vi "Big_LED_control.vi"() -> ()   [LabVIEW 2018]
uses:
  <instrlib>/niDCPower/nidcpower.llb/niDCPower Source Mode.ctl
  <instrlib>/niDCPower/nidcpower.llb/niDCPower Output Function.ctl
  AT lib/AmateurStepperMotor.dll
  <instrlib>/niDMM/nidmm.llb/niDMM Function.ctl
  <instrlib>/niDMM/nidmm.llb/niDMM Resolution in Digits.ctl
  <vilib>/Instr/_visa.llb/VISA Configure Serial Port (Instr).vi
  <instrlib>/niDMM/nidmm.llb/niDMM Configure Measurement Digits.vi
panel:
  in  "Go To 2":dbl
  in  "Погнали! 2":bool
  in  "HoldOn 2":bool
  in  "Tab Control 2":enum32{"Шаговик и офир", "Служебная область"}(tab)
  in  "milliseconds to wait":u32=1000
  in  "Go To":dbl
  out "Ophir 1 Char":dbl(graph)=0.02
  in  "DecelerationTime, s":dbl=0.3
  in  "AccelerationTime, s":dbl=0.3
  in  "HoldOn":bool
  in  "Ophir 1 units":string(combo)="1000" caption="Units"
  out "Ophir 1 Over Range":bool caption="Over Range"
  out "Ophir 1 Optical Power":dbl=0.02 caption="Power" format="%#_4g"
  out "Ophir 1 MAX":dbl=0.030000000000000002 caption="MAX" format="%#_5g"
  in  "Ophir 1 Clear":bool caption="Clear"
  in  "StepMultiplicationFactor":dbl=50.0
  in  "StepDivisor":i32(ring)=8 items=["D1"=1, "D2"=2, "D4"=4, "D8"=8, "D16"=16, "D32"=32]
  in  "Speed":dbl=250.0
  in  "Погнали!":bool
  in  "Стоп GoTo":bool
  out "Готово":bool
  out "Position":dbl
  in  "Ophir 1 Info":u16(ring)=1 caption="Info" items=["Device : JUNO; s/n:903793", "Head : PD300R-3W   ; s/n:779628"]
  in  "new pos":dbl
  in  "set pos":bool
  out "Device Response":string="*\n"
  in  "Ophir 1 usb channel":i16 caption="usb channel"
  out "Ophir 1 dup Visa Session":refnum<visa-resource-name>="USB0::0x0BD3::0x0777::NI-VISA-60004::RAW" caption="dup Visa Session"
  in  "Ophir 1 Baud Rate (3:9600)":i16(ring)=3 caption="Baud Rate (3:9600)" items=["300", "1200", "4800", "9600", "19200", "38400"]
  out "Ophir 1 Real Optical Power":dbl=2e-05 format="%.6e"
  in  "Ophir 1 GPIB Address (10)":string="10" caption="GPIB Address (10)"
  in  "Ophir 1 Port Number (default 2)":i16=1 caption="Port Number (default 2)" min=0 max=20
  in  "Ophir 1 Select Communication Protocol":u16(ring) caption="Select Communication Protocol" items=["USB", "RS232", "GPIB"]
  out "Ophir 1 error out":errorcluster caption="error out"
  in  "Ophir 1 error in (no error)":errorcluster caption="error in (no error)"
  in  "Ophir 1 Wait":u32=100 caption="Wait"
  out "IsOpen":bool=TRUE
  out "Ophir 1 Initialization":bool=TRUE caption="Initialization"
  in  "Tab Control":T1(tab)
  in  "POWER":bool
  in  "Стоп":bool=TRUE
  in  "Resource Name":refnum<k15>="PXI1Slot2" caption="Источник питания"
  in  "Амперметр":refnum<k15>="PXI1Slot4" caption="NI DMM 1"
  in  "V_MB, V":dbl=2.0 caption="voltage level" format="%_6p"
  in  "curlim_V_MB, A":dbl=0.3 caption="current limit" format="%_6p"
  out "chart_0":dbl(graph)=-0.00019003121552656476 caption="Waveform Chart 5"
  in  "voltlim_I_LED, V":dbl=2.0 caption="current limit" min=0.01 format="%_6p"
  in  "I_LED, A":dbl=0.005 caption="voltage level" format="%_6p"
  out "chart_1":dbl(graph)=-0.00011794146773492402 caption="Waveform Chart 5"
  out "Current Char":dbl(graph)=0.004513189196586609
  in  "Arduino":refnum<visa-resource-name>="COM14"
  in  "Сегменты":bool[](array[boolean])=[FALSE, FALSE, FALSE, FALSE, FALSE, FALSE, FALSE, FALSE, FALSE, FALSE, FALSE, FALSE, FALSE, FALSE, FALSE, FALSE, FALSE, FALSE]
  in  "Вольтметр":refnum<k15>="PXI1Slot5" caption="NI DMM 1"
  out "Voltage Char":dbl(graph)=0.015767553821206093
  in  "Port Name":string="COM4" caption="Порт шаговика"
  in  "wave_lenght":string="600"
  in  "Промер":bool caption="Промер сегмента"
  in  "NI DMM 1 Voltage Range 4":string(combo)="-1" caption="Range"
  in  "NI DMM 1 units 4":string(combo)="1" caption="Units"
  out "Voltage":dbl=0.015767553821206093 format="%_6g"
  in  "NI DMM 1 Current Range 3":string(combo)="1" caption="Range"
  in  "NI DMM 1 units 3":string(combo)="1000" caption="Units"
  out "Current":dbl=0.004513189196586609 format="%_6g"
  out "voltmes_V_MB, V":dbl=-0.00019003121552656476 caption="measurement" format="%_6g"
  out "curmes_V_MB, A":dbl=4.978853713564661e-05 caption="measurement" format="%_6g"
  out "curmes_I_LED, A":dbl=4.978853713564661e-05 caption="measurement" format="%_6g"
  out "voltmes_I_LED, V":dbl=-0.00011794146773492402 caption="measurement" format="%_6g"
  out "Разряд":dbl
  out "+/-":bool
  out "Power off":bool=TRUE
  in  "Command":string="Cathode"
  in  "Записать":bool
  out "measure output file refnum":refnum<file>
  out "Voltage, V":dbl=0.015767553821206093 caption="Measurement" format="%.5f"
  out "Current, A":dbl=4.513189196586609e-06 caption="Measurement" format="%.5f"
  out "Тип индикатора":string="Cathode"
  out "chart_2":dbl(graph)=-0.000179732680132088
  in  "V_RES, V":dbl caption="voltage level" format="%_6p"
  out "curmes_V_RES, A":dbl=5.996099535583298e-05 caption="measurement" format="%_6g"
  in  "curlim_V_RES, A":dbl=0.1 caption="current limit" min=0.01 format="%_6p"
  in  "measure path":path=path "D:/NI LabVIEW/MultiOpto/MultiOpto_1.2/Logs/SEL"
  out "Enum":enum16{"Exit", "4", "Промер", "2", "1"}(ring)
  out "№ об-ца":dbl=1.0
  out "Темп-ра":dbl=1.0
  out "Сегмент":string
  out "voltmes_V_RES, V":dbl=-0.000179732680132088 caption="measurement" format="%_6g"
  in  "current level range":dbl=0.001 format="%#.6p"
  # "Шаговик"
  # "Офир"
  # "Шаговик"
  # "Офир"
  # "position - это значение абсолютное"
  # "j"
  # "c"
  # "d"
  # "e"
  # "g"
  # "h"
  # "a"
  # "b"
  # "f"
  # "k"
  # "L"
  # "m"
  # "n"
  # "p"
  # "dp"
  # "all"
  # "V_MB 5 В\nогрничение 300 м\n\nV_LED 2,1 В\nограничение 200 м"
  # "единицы мА\nrange 1 А"
  # "1. каждый сегмент включаем по отдельности, резистором постраиваем ток до 10 мА\n2. напряжение V_LED при этом не меняется\n3. в такоом положении промеряем сегменты по отдельности\n4. для промера всего индикатора сразу подстраиваем напряжение при неизменном положении резисторов\n5. ток всех индикаторов = ток одного сегмента (10 мА) * число сегментов (15)\n6. добиваемся этого увеличением V_LED"
  # "единицы В\nrange AUTO"
  # "регклировка суммарного тока через индикатор"
  # "24.063\n\n     I          U\n20 мА  1.3 В\n20 мА  1.4 В\n 7 мА   1.15 В"
  # "24.064\n\n     I          U\n10 мА  2 В\n10 мА  2.15 В\n 7 мА   1.9 В"
  # "автоматизировать подбор напряжения по известному максимальному напряжению и току. ОС по току сегмента"
  # "Р1:  +25°C\nР2:  - 60°C\nР3:  +85°C"
  # "регулировать ток в зависимости от температуры.\nс ростом температуры растет ток.\nпид-регулятор??"
  # "0. ввести номер образца\n1. включить нужный сегмент\n2. ввести его в поле справа\n3. вести температуру в поле слева\n4. нажать кнопку \"промер сегмента\""
  # "\"опрашивать кнопки не чаще, чем раз в секунду. сейчас кликать можно чаще, они загорятся, но ничего не произойдет\""
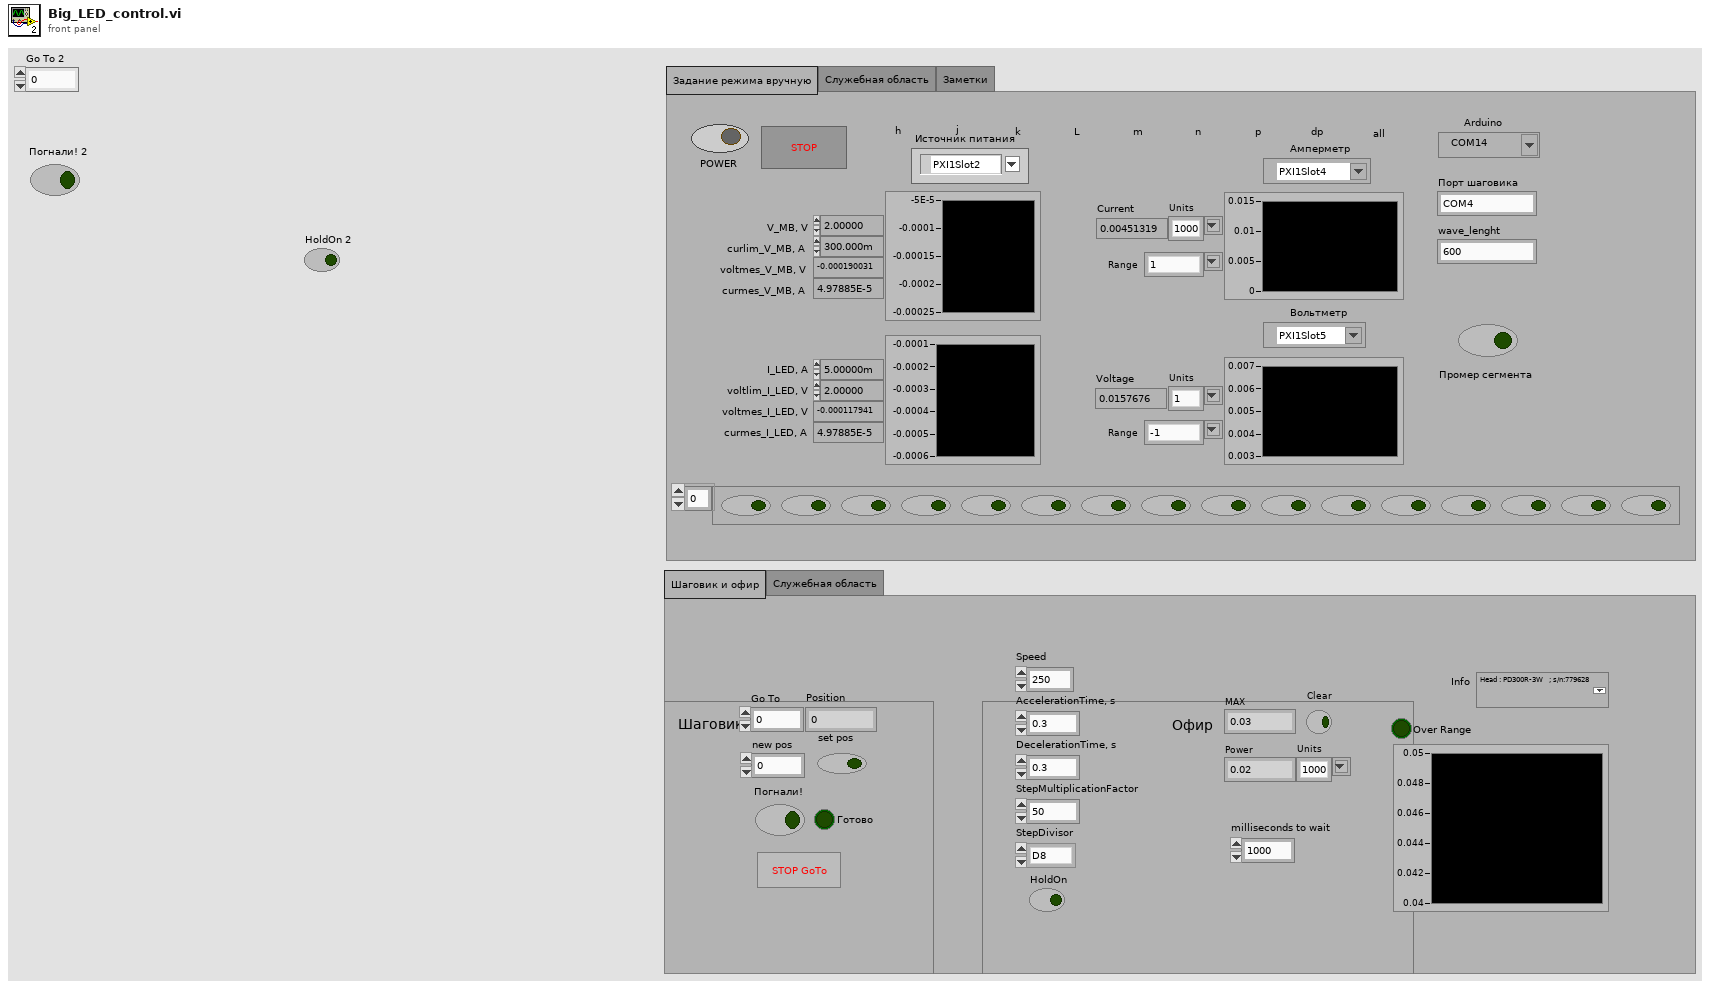
[diagram p1: front panel]
types:
  T1 = enum32{"Задание режима вручную", "Служебная область", "Заметки"}
  T2 = enum16{"open", "replace", "create", "open or create", "replace or create", "replace or create with confirmation"}
  T3 = typedef "niDCPower Output Function.ctl" = i32
  T4 = typedef "niDCPower Source Mode.ctl" = i32
  T5 = typedef "niDMM Function.ctl" = enum16{"DC Volts", "AC Volts", "DC Current", "AC Current", "2-wire Resistance", "4-wire Resistance", "Diode", "Frequency", "Period", "AC Volts DC Coupled", "Capacitance", "Inductance", "Temperature"}
  T6 = typedef "niDMM Resolution in Digits.ctl" = dbl
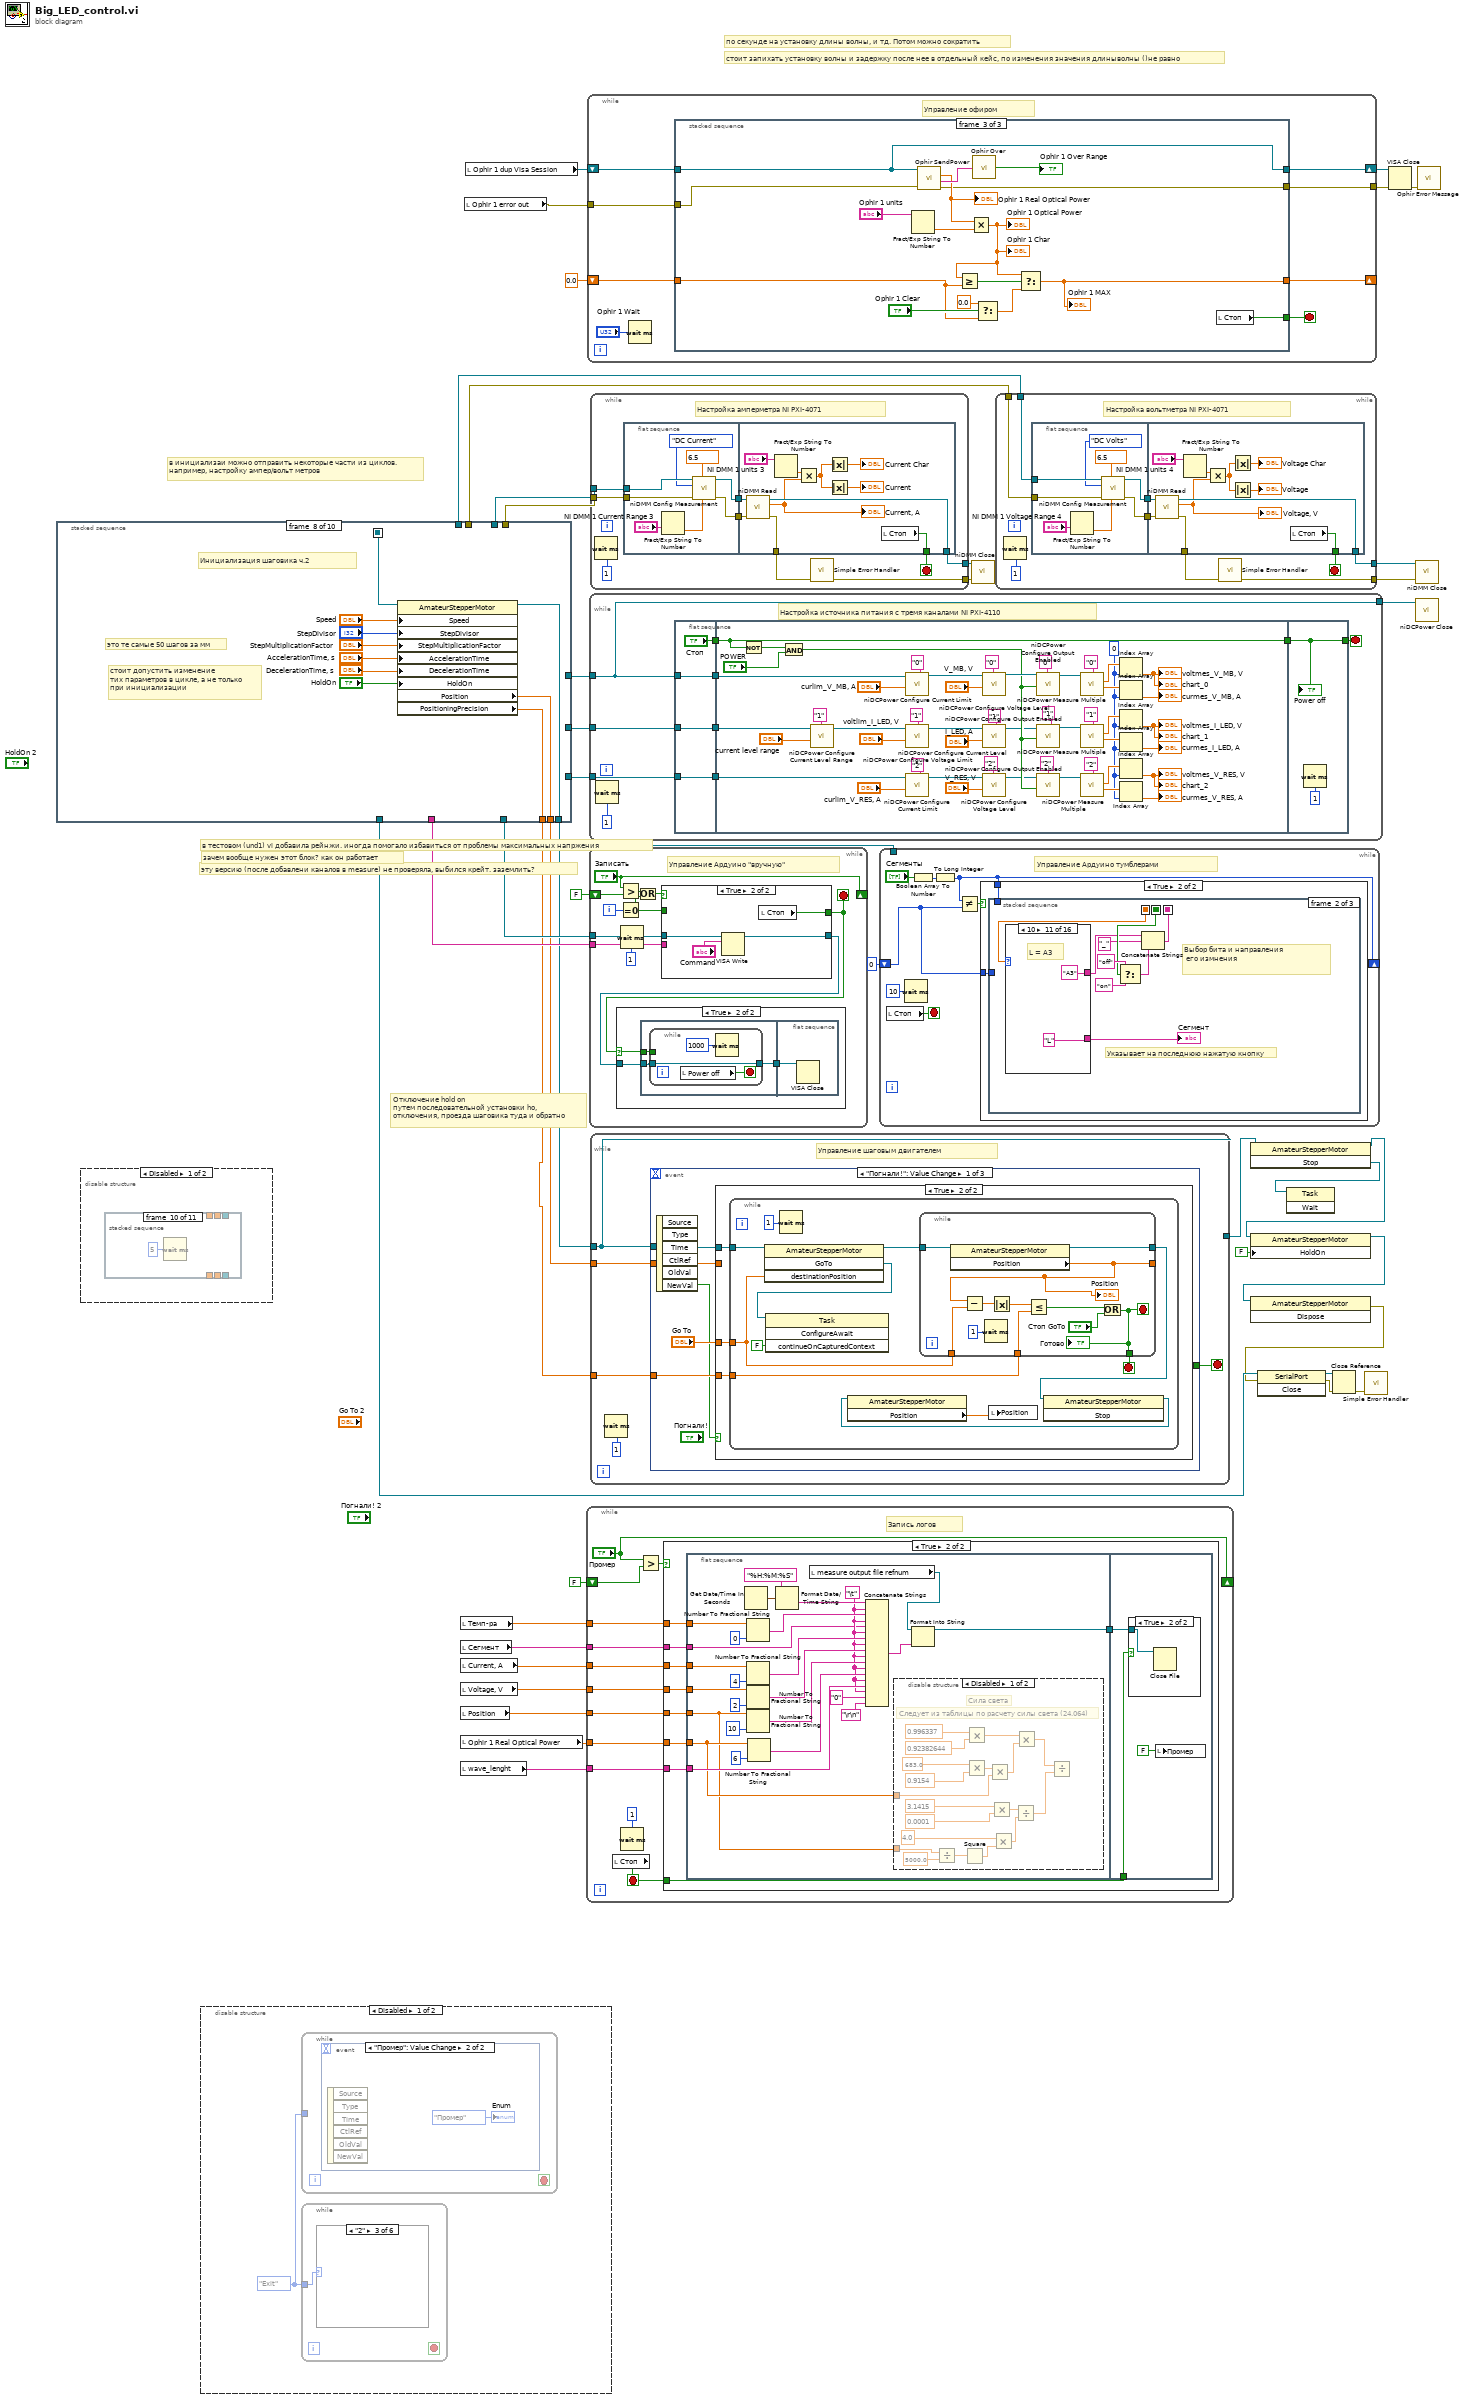
[diagram p0: block diagram]
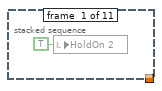
[diagram p2: hidden frame]
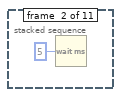
[diagram p3: hidden frame]
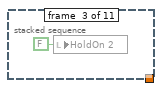
[diagram p4: hidden frame]
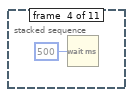
[diagram p5: hidden frame]
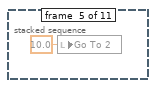
[diagram p6: hidden frame]
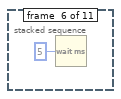
[diagram p7: hidden frame]
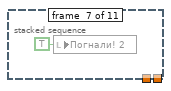
[diagram p8: hidden frame]
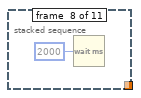
[diagram p9: hidden frame]
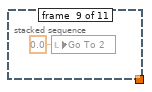
[diagram p10: hidden frame]
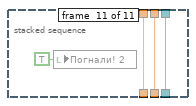
[diagram p11: hidden frame]
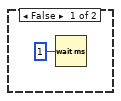
[diagram p13: hidden frame]
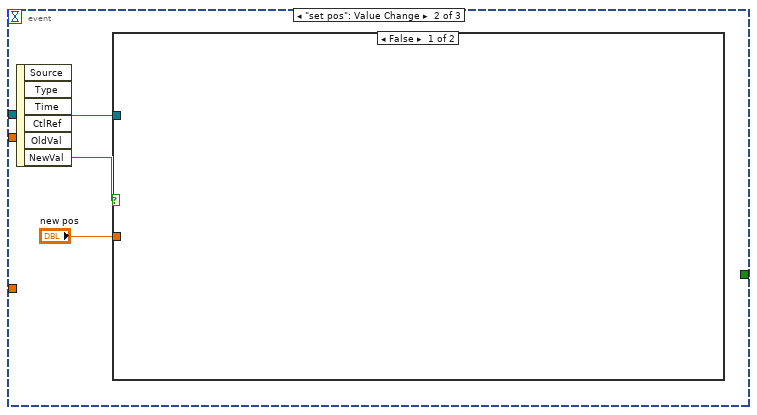
[diagram p14: hidden frame]
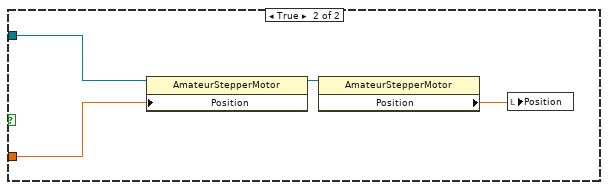
[diagram p15: hidden frame]
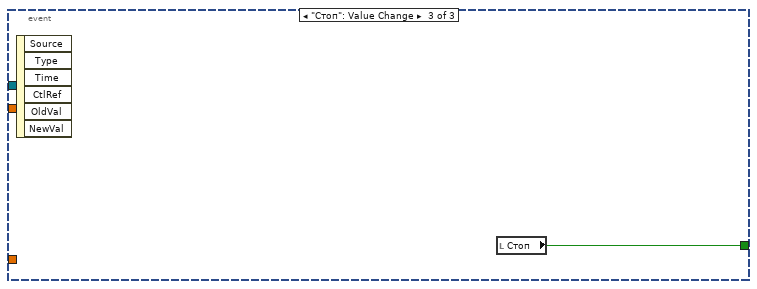
[diagram p16: hidden frame]
diagram:
  # "эту версию (после добавлени каналов в measure) не проверяла, выбился крейт. заземлить?"
  # "зачем вообще нужен этот блок? как он работает"
  # "в тестовом (und1) vi добавила рейнжи. иногда помогало избавиться от проблемы максимальных напржения"
  # "Отключение hold on\nпутем последовательной установки ho, \nотключения, проезда шаговика туда и обратно"
  # "в инициализаи можно отправить некоторые части из циклов.\nнапример, настройку ампер/вольт метров"
  # "стоит запихать установку волны и задержку после нее в отдельный кейс, по изменения значения длиныволны ()не равно"
  # "по секунде на установку длины волны, и тд. Потом можно сократить"
  n1 = stacked-sequence {
    seq-local: [_ _ _ _ _ _ w114 _ _ _] -> [_ _ _ _ _ _ _ w123 _ _]
    tunnel: [_ _ _ w61 _ _ _ _ _ _] -> w31
    tunnel: [_ w55 _ _ _ _ _ _ _ _] -> w43
    tunnel: [_ w54 _ _ _ _ _ _ _ _] -> w42
    tunnel: [_ _ _ _ w81 _ _ _ _ _] -> w39
    tunnel: [_ _ _ _ _ _ _ _ _ w161] -> w38
    tunnel: [_ _ w58 _ _ _ _ _ _ _] -> w37
    tunnel: [_ _ w57 _ _ _ _ _ _ _] -> w36
    tunnel: [_ _ _ _ _ _ _ w126 _ _] -> w1
    tunnel: [_ _ _ _ _ _ _ w124 _ _] -> w2
    tunnel: [_ _ _ _ _ _ _ w125 _ _] -> w3
    tunnel: [_ _ _ _ _ _ w104 _ _ _] -> w25
    tunnel: [_ _ _ w60 _ _ _ _ _ _] -> w8
    tunnel: [_ _ _ w59 _ _ _ _ _ _] -> w4
    frame #0 {
      w49 = 0.0 ("currentmes_2")
      w50 = FALSE ("Стоп")
      # "ch 1"
      # "Обнуление переменных"
      n2 = local write "POWER"(w50) -> ()
      n3 = local write "Стоп"(w50) -> ()
      n4 = local write "+/-"(w50) -> ()
      n5 = local write "Погнали!"(w50) -> ()
      n6 = local write "Готово"(w50) -> ()
      n7 = local write "Стоп GoTo"(w50) -> ()
      n8 = local write "Speed"(250.0 ("Speed")) -> ()
      n9 = local write "StepMultiplicationFactor"(50.0 ("StepMultiplicationFactor")) -> ()
      n10 = local write "AccelerationTime, s"(0.3 ("AccelerationTime, s")) -> ()
      n11 = local write "DecelerationTime, s"(0.3 ("DecelerationTime, s")) -> ()
      n12 = local write "Go To"(w49) -> ()
      n13 = local write "curmes_V_MB, A"(w49) -> ()
      n14 = local write "curmes_V_RES, A"(w49) -> ()
      n15 = local write "Current"(w49) -> ()
      n16 = local write "Разряд"(w49) -> ()
      n17 = local write "voltmes_I_LED, V"(w49) -> ()
      n18 = local write "Сегменты"(bool[] [FALSE, FALSE, FALSE, FALSE, FALSE, FALSE, FALSE, FALSE, FALSE, FALSE, FALSE, FALSE, FALSE, FALSE, FALSE, FALSE, FALSE, FALSE] ("Сегменты")) -> ()
      n19 = local write "current level range"(0.001 ("current level range")) -> ()
      n20 = local write "Command"("zero" ("Command 2")) -> ()
    }
    frame #1 {
      # "Инициализация амперметра"
      n21 = call <instrlib>:"niDMM Initialize.vi"("Instrument Descriptor"="Амперметр") -> ("error out"=w55:errorcluster, "instrument handle out"=w54:refnum<k15>)  [unwired: 9 in]
    }
    frame #2 {
      # "Инициализация вольтметра"
      n22 = call <instrlib>:"niDMM Initialize.vi"("Instrument Descriptor"="Вольтметр") -> ("error out"=w57:errorcluster, "instrument handle out"=w58:refnum<k15>)  [unwired: 9 in]
    }
    frame #3 {
      w66 = T3 1006 items=["DC Voltage"=1006, "DC Current"=1007, "Pulse Voltage"=1049, "Pulse Current"=1050] ("output function")
      w70 = T3 1007 items=["DC Voltage"=1006, "DC Current"=1007, "Pulse Voltage"=1049, "Pulse Current"=1050] ("output function")
      w71 = T3 1006 items=["DC Voltage"=1006, "DC Current"=1007, "Pulse Voltage"=1049, "Pulse Current"=1050] ("output function")
      w74 = T4 1020 items=["Single Point"=1020, "Sequence"=1021] ("source mode")
      # "Инициализация источника питания"
      n23 = call <instrlib>:"niDCPower Initialize.vi"("resource name"="Resource Name") -> ("instrument handle out"=w75:refnum<k15>)  [unwired: 3 in, 7 out]
      n24 = call <instrlib>:"niDCPower Configure Source Mode.vi"("source mode"=w74, "instrument handle"=w75) -> ("instrument handle out"=w65:refnum<k15>)  [unwired: 1 in, 8 out]
      n25 = call <instrlib>:"niDCPower Configure Output Function.vi"("output function"=w70, "channel name"="1", "instrument handle"=w65) -> ("instrument handle out"=w72:refnum<k15>)  [unwired: 7 in, 1 out]
      n26 = call <instrlib>:"niDCPower Configure Output Function.vi"("output function"=w66, "channel name"="2", "instrument handle"=w65) -> ("instrument handle out"=w67:refnum<k15>)  [unwired: 7 in, 1 out]
      n27 = call <instrlib>:"niDCPower Configure Output Function.vi"("output function"=w71, "channel name"="0", "instrument handle"=w65) -> ("instrument handle out"=w73:refnum<k15>)  [unwired: 7 in, 1 out]
      n28 = call <instrlib>:"niDCPower Configure Voltage Level.vi"("voltage level"=0.0, "channel name"="2", "instrument handle"=w67) -> ("instrument handle out"=w59:refnum<k15>)  [unwired: 7 in, 1 out]
      n29 = call <instrlib>:"niDCPower Configure Voltage Level.vi"("voltage level"=0.0, "channel name"="0", "instrument handle"=w73) -> ("instrument handle out"=w61:refnum<k15>)  [unwired: 7 in, 1 out]
      n30 = call <instrlib>:"niDCPower Configure Current Level.vi"("current level"=0.01, "channel name"="1", "instrument handle"=w72) -> ("instrument handle out"=w60:refnum<k15>)  [unwired: 7 in, 1 out]
    }
    frame #4 {
      # "Инициализация Ардуино"
      n31 = call-poly "VISA Configure Serial Port"("VISA resource name"="Arduino", "baud rate (9600)"=u32 9600) -> ("VISA resource name out"=w81:refnum<visa-resource-name>)  [unwired: 12 in, 1 out]
    }
    frame #5 {
      # "Инициализация офира"
      n32 = call "Ophir InitCom.vi"("GPIB Address (default 10)"="Ophir 1 GPIB Address (10)", "Communication (default USB 0)"="Ophir 1 Select Communication Protocol", "USB Channel number (default 0)"="Ophir 1 usb channel", "Port Number (default 2)"="Ophir 1 Port Number (default 2)", "error in (no error)"="Ophir 1 error in (no error)", "Baud Rate (3:9600)"="Ophir 1 Baud Rate (3:9600)") -> ("dup Visa Session"=w90:refnum<visa-resource-name>, "error out"=w89:errorcluster)  [unwired: 1 out]
      n33 = call "Ophir InstrInfo.vi"("Visa Session"=w90, "error in (no error)"=w89) -> ("dup Visa Session"=w102:refnum<visa-resource-name>, "Instrument Info"=w84:string, "error out"=w100:errorcluster)
      n34 = call "Ophir HeadInfo.vi"("Visa Session"=w102, "error in (no error)"=w100) -> ("error out"=w99:errorcluster, "dup Visa Session"=w101:refnum<visa-resource-name>, "Head Info"=w98:string)  [unwired: 6 out]
      n35 = call "Ophir InfoStrings.vi"("error in (no error)"=w99, "Head Info"=w98, "Instrument Info"=w84) -> ("error out"=w97:errorcluster, "Strings Array"=w96:string[])
      n36 = property on="Ophir 1 Info" class="Ring (strict)"("Strings []"=w96) -> ()  [unwired: 2 in, 2 out]
      n37 = call "Ophir ConfigDevice.vi"("Visa Session"=w101, "Measure Choice (0:Power)"=u16 0, "error in (no error)"=w97) -> ("dup Visa Session"=→"Ophir 1 dup Visa Session":refnum<visa-resource-name>, "OK ?"=→"Ophir 1 Initialization":bool, "error out"=→"Ophir 1 error out":errorcluster)  [unwired: 1 out]
    }
    frame #6 {
      w108 = 100 ("WriteTimeout")
      w113 = 1 items=["None", "One", "Two", "OnePointFive"] ("stopBits")
      w110 = 0 items=["None", "Odd", "Even", "Mark", "Space"] ("parity")
      # "убрали открытие порта. шаговик его и так сам откроет"
      # "Инициализация шаговика ч.1"
      n38 = constructor class="SerialPort"("portName"="Port Name", "baudRate"=57600, "parity"=w110, "dataBits"=8, "stopBits"=w113) -> (reference out=w107:refnum<k24>, error out=w106:errorcluster)  [unwired: 3 in, 6 out]
      n39 = property class="SerialPort"(reference=w107, error in=w106, "WriteTimeout"=w108, "ReadTimeout"=w108) -> (reference out=w104:refnum<k24>)  [unwired: 1 out]
      n40 = constructor class="AmateurStepperMotor"("serialPort"=w104) -> (reference out=w114:refnum<k24>, error out=w105:errorcluster)  [unwired: 3 in, 2 out]
      n41 = flat-sequence {
        tunnel: w105 -> [_]
        tunnel: w104 -> [w116]
        frame #0 {
          n42 = property class="SerialPort"(reference=w116) -> ("IsOpen"=→"IsOpen":bool)  [unwired: 1 in, 2 out]
        }
      }
    }
    frame #7 {
      # "стоит допустить изменение\nтих параметров в цикле, а не только \nпри инициализации"
      # "это те самые 50 шагов за мм"
      # "Инициализация шаговика ч.2"
      n43 = property class="AmateurStepperMotor"(reference=w123, "Speed"="Speed", "StepDivisor"="StepDivisor", "StepMultiplicationFactor"="StepMultiplicationFactor", "AccelerationTime"="AccelerationTime, s", "DecelerationTime"="DecelerationTime, s", "HoldOn"="HoldOn") -> (reference out=w126:refnum<k24>, "Position"=w124:dbl, "PositioningPrecision"=w125:dbl)  [unwired: 1 in, 1 out]
    }
    frame #8 {
      w132 = "\t"
      # "Инициализация логов"
      n44 = local read "№ об-ца"() -> (w128:dbl)
      n45 = Number To Fractional String(number=w128, precision (6)=i16 0) -> (F-format string=w129:string)  [unwired: 2 in]
      n46 = Get Date/Time In Seconds() -> (seconds since 1Jan1904=w150:timestamp)
      n47 = Build Path(base path="measure path", name or relative path=w129) -> (appended path=w146:path)
      n48 = call <vilib>:"Check if File or Folder Exists.vi"("path"=w146) -> ("file or folder exists?"=w147:bool, "dup path"=w148:path)  [unwired: 8 in, 1 out]
      n49 = Format Date/Time String(time format string (%c)="MES %d %m %y %H.%M.%S", seconds (now)=w150) -> (date/time string=w151:string)  [unwired: 1 in]
      n50 = case shown="False" w147 {
        tunnel: w148 -> [w159 w160]
        tunnel: [w158 w160] -> w149
        frame False {
          n51 = Create Folder(path (use dialog)=w159) -> (created path=w158:path)  [unwired: 2 in, 2 out]
        }
        frame True {
        }
      }
      n52 = Concatenate Strings(w151, ".xls" ("string")) -> (w152:string)
      n53 = Build Path(base path=w149, name or relative path=w152) -> (appended path=w153:path)
      n54 = Open/Create/Replace File(file path (use dialog)=w153, operation (0:open)=T2."open or create", access (0:read/write)=enum16{"read/write", "read-only", "write-only"}."read/write") -> (refnum out=w154:refnum<file>)  [unwired: 3 in, 2 out]
      n55 = Set File Position(refnum=w154, from (0:start)=enum16{"start", "end", "current"}."end") -> (refnum out=w156:refnum<file>)  [unwired: 2 in, 1 out]
      n56 = Format Into String(initial string=w156, "Time" ("string"), w132, "Temperature, C" ("string"), w132, "Segment" ("string"), w132, "Current, mA" ("string"), w132, "Voltage, V" ("input 7"), w132, "Distance, m" ("string"), w132, "Power, W " ("string"), w132, "Wavelenght, nm" ("input 17"), w132, "Candlepower, kd" ("string"), "\r\n") -> (resulting string=→"measure output file refnum":refnum<file>)  [unwired: 2 in, 1 out]
    }
    frame #9 {
      # "Begin VI: ОК или ОА?"
      n57 = disable-structure shown="Disabled" {
        disable-tunnel: [w164 _] -> w161
        frame Disabled {
          n58 = call "Begin.vi"() -> ("Темп-ра"=→"Темп-ра":dbl, "№ об-ца"=→"№ об-ца":dbl, "String"=w164:string)  [unwired: 6 in]
          "Тип индикатора" <- w164
          n59 = local write "Command"(w164) -> ()
        }
        frame Enabled {
        }
      }
    }
  }
  n60 = disable-structure shown="Disabled" {
    frame Disabled {
      n61 = stacked-sequence {
        tunnel: _ -> [_ _ _ _ _ _ _ _ _ _ w177]
        tunnel: [_ _ _ _ _ _ _ _ _ _ w177] -> _
        tunnel: _ -> [_ _ _ _ _ _ _ _ _ _ w176]
        tunnel: [_ _ _ _ _ _ _ _ _ _ w176] -> _
        tunnel: [_ _ _ _ _ _ _ _ _ _ w175] -> _
        tunnel: _ -> [_ _ _ _ _ _ _ _ _ _ w175]
        frame #0 {
          n62 = local write "HoldOn 2"(TRUE ("HoldOn")) -> ()
        }
        frame #1 {
          n63 = Wait (ms)(milliseconds to wait=u32 5) -> ()  [unwired: 1 out]
        }
        frame #2 {
          n64 = local write "HoldOn 2"(FALSE ("HoldOn")) -> ()
        }
        frame #3 {
          n65 = Wait (ms)(milliseconds to wait=u32 500) -> ()  [unwired: 1 out]
        }
        frame #4 {
          n66 = local write "Go To 2"(10.0 ("Go To")) -> ()
        }
        frame #5 {
          n67 = Wait (ms)(milliseconds to wait=u32 5) -> ()  [unwired: 1 out]
        }
        frame #6 {
          n68 = local write "Погнали! 2"(TRUE ("Погнали!")) -> ()
        }
        frame #7 {
          n69 = Wait (ms)(milliseconds to wait=u32 2000) -> ()  [unwired: 1 out]
        }
        frame #8 {
          n70 = local write "Go To 2"(0.0 ("Go To")) -> ()
        }
        frame #9 {
          n71 = Wait (ms)(milliseconds to wait=u32 5) -> ()  [unwired: 1 out]
        }
        frame #10 {
          n72 = local write "Погнали! 2"(TRUE ("Погнали!")) -> ()
        }
      }
    }
    frame Enabled {
    }
  }
  n73 = disable-structure shown="Disabled" {
    frame Disabled {
      w179 = enum16{"Exit", "4", "Промер", "2", "1"}."Exit"
      n74 = while {
        tunnel: w179 -> [w180]
        stop <- _ stop-if-true
        n75 = case shown="\"2\"" w180 {
          frame "Exit", Default {
          }
          frame "4" {
          }
          frame "2" {
          }
          frame "2" {
          }
          frame "1" {
          }
          frame "Промер" {
          }
        }
      }
      n76 = while {
        tunnel: w179 -> [_]
        stop <- _ stop-if-true
        n77 = event shown="[1] \"Промер\": Value Change" {
          selector: _ -> [_ _]
          dyn-events: _ -> [_ _]
          timeout: _ -> [_ _]
          event Timeout {
            n78 = event-data() -> ()  [unwired: 1 in, 3 out]
          }
          event "Промер": Value Change {
            n79 = event-data() -> ()  [unwired: 1 in, 6 out]
            "Enum" <- enum16{"Exit", "4", "Промер", "2", "1"}."Промер" ("Enum")
          }
        }
      }
    }
    frame Enabled {
    }
  }
  n80 = local read "Темп-ра"() -> (w6:dbl)
  n81 = local read "Сегмент"() -> (w5:string)
  n82 = local read "Current, A"() -> (w24:dbl)
  n83 = local read "Voltage, V"() -> (w23:dbl)
  n84 = local read "Position"() -> (w22:dbl)
  n85 = local read "Ophir 1 Real Optical Power"() -> (w21:dbl)
  n86 = local read "wave_lenght"() -> (w20:string)
  n87 = local read "Ophir 1 error out"() -> (w29:errorcluster)
  n88 = local read "Ophir 1 dup Visa Session"() -> (w30:refnum<visa-resource-name>)
  n89 = while {
    tunnel: w24 -> [w193]
    tunnel: w23 -> [w192]
    tunnel: w22 -> [w191]
    tunnel: w21 -> [w190]
    tunnel: w20 -> [w189]
    shift-right: ["Промер"] -> _
    shift-left: FALSE ("Промер сегмента") -> [w186]
    tunnel: w6 -> [w183]
    tunnel: w5 -> [w182]
    stop <- w184 stop-if-true
    # "Запиcь логов"
    n90 = local read "Стоп"() -> (w184:bool)
    n91 = Wait (ms)(milliseconds to wait=u32 1) -> ()  [unwired: 1 out]
    n92 = Greater?(x="Промер", y=w186) -> (0:w187:bool)
    n93 = case shown="True" w187 {
      tunnel: w193 -> [_ w202]
      tunnel: w192 -> [_ w201]
      tunnel: w191 -> [_ w198]
      tunnel: w190 -> [_ w199]
      tunnel: w189 -> [_ w200]
      tunnel: w184 -> [_ w196]
      tunnel: w183 -> [_ w195]
      tunnel: w182 -> [_ w194]
      frame False {
      }
      frame True {
        n94 = flat-sequence {
          tunnel: w202 -> [w220]
          tunnel: w201 -> [w219]
          tunnel: w200 -> [w217]
          tunnel: w199 -> [w216]
          tunnel: w198 -> [w215]
          tunnel: [w210] -> w197
          tunnel: w195 -> [w209]
          tunnel: w194 -> [w203]
          tunnel: w197 -> [w250]
          tunnel: w196 -> [w249]
          frame #0 {
            w205 = "\t"
            n95 = Get Date/Time In Seconds() -> (seconds since 1Jan1904=w228:timestamp)
            n96 = Number To Fractional String(number=w209, precision (6)=i16 0) -> (F-format string=w207:string)  [unwired: 2 in]
            n97 = Number To Fractional String(number=w220, precision (6)=i16 4) -> (F-format string=w223:string)  [unwired: 2 in]
            n98 = Number To Fractional String(number=w219, precision (6)=i16 2) -> (F-format string=w222:string)  [unwired: 2 in]
            n99 = Number To Fractional String(number=w215, precision (6)=i16 10) -> (F-format string=w221:string)  [unwired: 2 in]
            n100 = Number To Fractional String(number=w216, precision (6)=i16 6) -> (F-format string=w218:string)  [unwired: 2 in]
            n101 = Format Date/Time String(time format string (%c)="%H:%M:%S", seconds (now)=w228) -> (date/time string=w226:string)  [unwired: 1 in]
            n102 = local read "measure output file refnum"() -> (w224:refnum<file>)
            n103 = Concatenate Strings(w226, w205, w207, w205, w203, w205, w223, w205, w222, w205, w221, w205, w218, w205, w217, w205, "0" ("string"), "\r\n") -> (w225:string)
            n104 = disable-structure shown="Disabled" {
              disable-tunnel: w216 -> [w240 _]
              disable-tunnel: w215 -> [w230 _]
              frame Disabled {
                # "Сила света"
                # "Следует из таблицы по расчету силы света (24.064)"
                n105 = Divide(x=w230, y=5000.0) -> (x/y=w232:dbl)
                n106 = Square(x=w232) -> (x^2=w231:dbl)
                n107 = Multiply(x=0.996337, y=0.92382644) -> (x*y=w245:dbl)
                n108 = Multiply(x=683.0, y=0.9154) -> (x*y=w241:dbl)
                n109 = Multiply(x=w241, y=w240) -> (x*y=w239:dbl)
                n110 = Multiply(x=3.1415, y=0.0001) -> (x*y=w235:dbl)
                n111 = Multiply(x=4.0, y=w231) -> (x*y=w234:dbl)
                n112 = Divide(x=w235, y=w234) -> (x/y=w236:dbl)
                n113 = Multiply(x=w245, y=w239) -> (x*y=w244:dbl)
                n114 = Divide(x=w244, y=w236) -> ()  [unwired: 1 out]
              }
              frame Enabled {
              }
            }
            n115 = Format Into String(initial string=w224, w225) -> (resulting string=w210:refnum<file>)  [unwired: 2 in, 1 out]
          }
          frame #1 {
            n116 = case shown="True" w249 {
              tunnel: w250 -> [_ w251]
              frame False {
              }
              frame True {
                n117 = Close File(refnum=w251) -> ()  [unwired: 1 in, 2 out]
              }
            }
            n118 = local write "Промер"(FALSE ("Промер")) -> ()
          }
        }
      }
    }
  }
  n119 = while {
    tunnel: w29 -> [w258]
    shift-right: [w254] -> _
    shift-left: 0.0 ("t") -> [w257]
    shift-right: [w255] -> w18
    shift-left: w30 -> [w259]
    tunnel: [w253] -> w17
    stop <- w252 stop-if-true
    # "Управление офиром"
    n120 = Wait (ms)(milliseconds to wait="Ophir 1 Wait") -> ()  [unwired: 1 out]
    n121 = stacked-sequence {
      tunnel: w259 -> [w263 _ w266]
      tunnel: w258 -> [w262 _ w268]
      tunnel: w257 -> [_ _ w269]
      tunnel: [_ _ w266] -> w255
      tunnel: [_ _ w270] -> w254
      tunnel: [_ _ w267] -> w253
      tunnel: [_ _ w265] -> w252
      frame #0 {
        n122 = call "light_setWaveLenght.vi"("error in (no error)"=w262, "Visa Session"=w263, "wave_lenght"="wave_lenght") -> ("Device Response"=→"Device Response":string)  [unwired: 6 in, 2 out]
      }
      frame #1 {
        n123 = Wait (ms)(milliseconds to wait="milliseconds to wait") -> ()  [unwired: 1 out]
      }
      frame #2 {
        n124 = Fract/Exp String To Number(string="Ophir 1 units") -> (number=w273:dbl)  [unwired: 3 in, 1 out]
        n125 = call "Ophir SendPower.vi"("Visa Session"=w266, "error in (no error)"=w268) -> ("Value Number"=w272:dbl, "Value String"=w279:string, "error out"=w267:errorcluster)  [unwired: 1 out]
        "Ophir 1 Real Optical Power" <- w272
        n126 = Multiply(x=w272, y=w273) -> (x*y=w276:dbl)
        "Ophir 1 Char" <- w276
        "Ophir 1 Optical Power" <- w276
        n127 = Greater Or Equal?(x=w276, y=w269) -> (x >= y?=w277:bool)
        n128 = call "Ophir Over.vi"("Value String"=w279) -> ("Overrange"=→"Ophir 1 Over Range":bool)
        n129 = Select(t=0.0, s="Ophir 1 Clear", f=w269) -> (s? t:f=w275:dbl)
        n130 = Select(t=w276, s=w277, f=w275) -> (s? t:f=w270:dbl)
        "Ophir 1 MAX" <- w270
        n131 = local read "Стоп"() -> (w265:bool)
      }
    }
  }
  n132 = while {
    tunnel: w31 -> [w287]
    tunnel: [w287] -> w40
    tunnel: w8 -> [w284]
    tunnel: w4 -> [w281]
    stop <- w283 stop-if-true
    # "Настройка источника питания с тремя каналами NI PXI-4110"
    n133 = Wait (ms)(milliseconds to wait=u32 1) -> ()  [unwired: 1 out]
    n134 = flat-sequence {
      tunnel: w287 -> [w294]
      tunnel: [w294] -> w289
      tunnel: ["Стоп"] -> w288
      tunnel: [w292] -> w285
      tunnel: w284 -> [w292]
      tunnel: [w291] -> w282
      tunnel: w281 -> [w291]
      tunnel: w289 -> [w340]
      tunnel: w288 -> [w344]
      tunnel: [w344] -> w286
      tunnel: w285 -> [w308]
      tunnel: w282 -> [w301]
      tunnel: [w346] -> w283
      tunnel: w286 -> [w346]
      frame #0 {
      }
      frame #1 {
        w309 = 0 ("index")
        n135 = Not(x=w344) -> (.not. x?=w343:bool)
        n136 = And(x=w343, y="POWER") -> (x .and. y?=w339:bool)
        n137 = call <instrlib>:"niDCPower Configure Current Level Range.vi"("current level range"="current level range", "channel name"="1", "instrument handle"=w308) -> ("instrument handle out"=w307:refnum<k15>)  [unwired: 7 in, 1 out]
        n138 = call <instrlib>:"niDCPower Configure Current Limit.vi"("current limit"="curlim_V_MB, A", "channel name"="0", "instrument handle"=w340) -> ("instrument handle out"=w330:refnum<k15>)  [unwired: 7 in, 1 out]
        n139 = call <instrlib>:"niDCPower Configure Voltage Limit.vi"("voltage limit"="voltlim_I_LED, V", "channel name"="1", "instrument handle"=w307) -> ("instrument handle out"=w334:refnum<k15>)  [unwired: 7 in, 1 out]
        n140 = call <instrlib>:"niDCPower Configure Current Limit.vi"("current limit"="curlim_V_RES, A", "channel name"="2", "instrument handle"=w301) -> ("instrument handle out"=w324:refnum<k15>)  [unwired: 7 in, 1 out]
        n141 = call <instrlib>:"niDCPower Configure Voltage Level.vi"("voltage level"="V_MB, V", "channel name"="0", "instrument handle"=w330) -> ("instrument handle out"=w341:refnum<k15>)  [unwired: 7 in, 1 out]
        n142 = call <instrlib>:"niDCPower Configure Current Level.vi"("current level"="I_LED, A", "channel name"="1", "instrument handle"=w334) -> ("instrument handle out"=w335:refnum<k15>)  [unwired: 7 in, 1 out]
        n143 = call <instrlib>:"niDCPower Configure Voltage Level.vi"("voltage level"="V_RES, V", "channel name"="2", "instrument handle"=w324) -> ("instrument handle out"=w325:refnum<k15>)  [unwired: 7 in, 1 out]
        n144 = call <instrlib>:"niDCPower Configure Output Enabled.vi"("output enabled"=w339, "channel name"="0", "instrument handle"=w341) -> ("instrument handle out"=w318:refnum<k15>)  [unwired: 7 in, 1 out]
        n145 = call <instrlib>:"niDCPower Configure Output Enabled.vi"("output enabled"=w339, "channel name"="1", "instrument handle"=w335) -> ("instrument handle out"=w311:refnum<k15>)  [unwired: 7 in, 1 out]
        n146 = call <instrlib>:"niDCPower Configure Output Enabled.vi"("output enabled"=w339, "channel name"="2", "instrument handle"=w325) -> ("instrument handle out"=w310:refnum<k15>)  [unwired: 7 in, 1 out]
        n147 = call <instrlib>:"niDCPower Measure Multiple.vi"("channel name"="0", "instrument handle"=w318) -> ("current measurements"=w316:dbl[], "voltage measurements"=w317:dbl[])  [unwired: 6 in, 2 out]
        n148 = call <instrlib>:"niDCPower Measure Multiple.vi"("channel name"="1", "instrument handle"=w311) -> ("current measurements"=w314:dbl[], "voltage measurements"=w315:dbl[])  [unwired: 6 in, 2 out]
        n149 = call <instrlib>:"niDCPower Measure Multiple.vi"("channel name"="2", "instrument handle"=w310) -> ("current measurements"=w312:dbl[], "voltage measurements"=w313:dbl[])  [unwired: 6 in, 2 out]
        n150 = Index Array(array=w317, index=w309) -> (element=→"chart_0" →"voltmes_V_MB, V":dbl)
        n151 = Index Array(array=w316, index=w309) -> (element=→"curmes_V_MB, A":dbl)
        n152 = Index Array(array=w315, index=w309) -> (element=→"chart_1" →"voltmes_I_LED, V":dbl)
        n153 = Index Array(array=w314, index=w309) -> (element=→"curmes_I_LED, A":dbl)
        n154 = Index Array(array=w313, index=w309) -> (element=→"chart_2" →"voltmes_V_RES, V":dbl)
        n155 = Index Array(array=w312, index=w309) -> (element=→"curmes_V_RES, A":dbl)
      }
      frame #2 {
        n156 = Wait (ms)(milliseconds to wait=u32 1) -> ()  [unwired: 1 out]
        "Power off" <- w346
      }
    }
  }
  n157 = while {
    tunnel: w39 -> [w354]
    shift-right: ["Записать"] -> _
    shift-left: FALSE ("Записать") -> [w356]
    tunnel: w38 -> [w352]
    i -> [w353]
    stop <- w347 stop-if-true
    # "Управление Ардуино \"вручную\""
    n158 = Greater?(x="Записать", y=w356) -> (0:w350:bool)
    n159 = Equal To 0?(x=w353) -> (x = 0?=w349:bool)
    n160 = Wait (ms)(milliseconds to wait=u32 1) -> ()  [unwired: 1 out]
    n161 = Or(x=w350, y=w349) -> (x .or. y?=w351:bool)
    n162 = case shown="True" w351 {
      tunnel: w354 -> [w368 w373]
      tunnel: [w369 w372] -> w347
      tunnel: w352 -> [_ _]
      tunnel: w349 -> [_ _]
      tunnel: [w368 w370] -> w348
      frame False {
        n163 = local read "Стоп"() -> (w369:bool)
      }
      frame True {
        n164 = VISA Write(VISA resource name=w373, write buffer="Command") -> (VISA resource name out=w370:refnum<visa-resource-name>)  [unwired: 1 in, 2 out]
        n165 = local read "Стоп"() -> (w372:bool)
      }
    }
    n166 = case shown="True" w347 {
      selector: w347 -> [_ w358]
      tunnel: w348 -> [_ w360]
      frame False {
      }
      frame True {
        n167 = flat-sequence {
          tunnel: w360 -> [w363]
          tunnel: [w362] -> w359
          tunnel: w358 -> [w361]
          tunnel: w359 -> [w367]
          frame #0 {
            n168 = while {
              tunnel: w363 -> [w366]
              tunnel: [w366] -> w362
              tunnel: w361 -> [_]
              stop <- w364 stop-if-true
              n169 = local read "Power off"() -> (w364:bool)
              n170 = Wait (ms)(milliseconds to wait=u32 1000) -> ()  [unwired: 1 out]
            }
          }
          frame #1 {
            n171 = VISA Close(VISA resource name=w367) -> ()  [unwired: 1 in, 1 out]
          }
        }
      }
    }
  }
  n172 = while {
    tunnel: [w380] -> w32
    tunnel: w42 -> [w378]
    tunnel: w43 -> [w377]
    tunnel: [w374] -> w33
    stop <- w376 stop-if-true
    # "Настройка амперметра NI PXI-4071"
    n173 = Wait (ms)(milliseconds to wait=u32 1) -> ()  [unwired: 1 out]
    n174 = flat-sequence {
      tunnel: [w387] -> w382
      tunnel: w378 -> [w385]
      tunnel: w377 -> [w389]
      tunnel: [w386] -> w381
      tunnel: w382 -> [w398]
      tunnel: w381 -> [w401]
      tunnel: [w397] -> w376
      tunnel: [w396] -> w374
      tunnel: [w395] -> w375
      frame #0 {
        w383 = T6 6.5 items=["3 1/2"=3.5, "4 1/2"=4.5, "5 1/2"=5.5, "6 1/2"=6.5, "7 1/2"=7.5] ("Resolution in Digits")
        n175 = Fract/Exp String To Number(string="NI DMM 1 Current Range 3") -> (number=w388:dbl)  [unwired: 3 in, 1 out]
        n176 = call-poly <instrlib>:"niDMM Config Measurement.vi"("Range"=w388, "Resolution in Digits"=w383, "error in (no error)"=w389, "Function"=niDMM_Function."DC Current" ("Measurement Type"), "instrument handle"=w385) -> ("error out"=w386:errorcluster, "instrument handle out"=w387:refnum<k15>)  [unwired: 5 in]
      }
      frame #1 {
        n177 = call <instrlib>:"niDMM Read.vi"("error in (no error)"=w401, "instrument handle"=w398) -> ("error out"=w395:errorcluster, "Measurement"=w391:dbl, "instrument handle out"=w396:refnum<k15>)  [unwired: 7 in]
        "Current, A" <- w391
        n178 = Fract/Exp String To Number(string="NI DMM 1 units 3") -> (number=w399:dbl)  [unwired: 3 in, 1 out]
        n179 = Multiply(x=w399, y=w391) -> (x*y=w392:dbl)
        n180 = Absolute Value(x=w392) -> (abs(x)=→"Current Char":dbl)
        n181 = Absolute Value(x=w392) -> (abs(x)=→"Current":dbl)
        n182 = local read "Стоп"() -> (w397:bool)
      }
    }
    n183 = call <vilib>:"Simple Error Handler.vi"("error in (no error)"=w375) -> ("error out"=w380:errorcluster)  [unwired: 1 in, 7 out]
  }
  n184 = while {
    tunnel: w1 -> [w403]
    tunnel: w3 -> [w405]
    tunnel: [w403] -> w7
    tunnel: w2 -> [w406]
    stop <- w402 stop-if-true
    # "Управление шаговым двигателем"
    n185 = Wait (ms)(milliseconds to wait=u32 1) -> ()  [unwired: 1 out]
    n186 = event shown="[0] \"Погнали!\": Value Change" {
      selector: _ -> [_ _ _]
      dyn-events: _ -> [_ _ _]
      timeout: _ -> [_ _ _]
      tunnel: w403 -> [w411 w439 _]
      tunnel: w406 -> [w410 _ _]
      tunnel: w405 -> [w409 _ _]
      tunnel: [_ _ w445] -> w402
      event "Погнали!": Value Change {
        n187 = event-data() -> ("NewVal"=w407:bool)  [unwired: 1 in, 5 out]
        n188 = case shown="True" w407 {
          tunnel: "Go To" -> [_ w415]
          tunnel: w411 -> [_ w414]
          tunnel: w410 -> [_ _]
          tunnel: w409 -> [_ w413]
          frame False {
            n189 = Wait (ms)(milliseconds to wait=u32 1) -> ()  [unwired: 1 out]
          }
          frame True {
            n190 = while {
              tunnel: w415 -> [w422]
              tunnel: w414 -> [w423]
              tunnel: w413 -> [w425]
              stop <- w426 stop-if-true
              n191 = invoke class="AmateurStepperMotor" method="GoTo"(reference=w423, "destinationPosition"=w422) -> (reference out=w418:refnum<k24>, "GoTo"=w421:refnum<k24>)  [unwired: 2 in, 2 out]
              n192 = invoke class="Task" method="ConfigureAwait"(reference=w421, "continueOnCapturedContext"=FALSE) -> ()  [unwired: 2 in, 4 out]
              n193 = Wait (ms)(milliseconds to wait=u32 1) -> ()  [unwired: 1 out]
              n194 = while {
                tunnel: [w427] -> _
                tunnel: [w429] -> w419
                tunnel: [w431] -> w426
                tunnel: w422 -> [w436]
                tunnel: w425 -> [w434]
                tunnel: w418 -> [w428]
                stop <- w431 stop-if-true
                n195 = property class="AmateurStepperMotor"(reference=w428) -> (reference out=w429:refnum<k24>, "Position"=w427:dbl)  [unwired: 1 in, 1 out]
                "Position" <- w427
                n196 = Subtract(x=w427, y=w436) -> (x-y=w437:dbl)
                n197 = Wait (ms)(milliseconds to wait=u32 1) -> ()  [unwired: 1 out]
                n198 = Absolute Value(x=w437) -> (abs(x)=w435:dbl)
                n199 = Less Or Equal?(x=w435, y=w434) -> (x <= y?=w433:bool)
                n200 = Or(x=w433, y="Стоп GoTo") -> (x .or. y?=w431:bool)
                "Готово" <- w431
              }
              n201 = invoke class="AmateurStepperMotor" method="Stop"(reference=w419) -> (reference out=w417:refnum<k24>)  [unwired: 2 in, 2 out]
              n202 = property class="AmateurStepperMotor"(reference=w417) -> ("Position"=w416:dbl)  [unwired: 1 in, 2 out]
              n203 = local write "Position"(w416) -> ()
            }
          }
        }
      }
      event "set pos": Value Change {
        n204 = event-data() -> ("NewVal"=w440:bool)  [unwired: 1 in, 5 out]
        n205 = case shown="False" w440 {
          tunnel: w439 -> [_ w444]
          tunnel: "new pos" -> [_ w443]
          frame False {
          }
          frame True {
            n206 = property class="AmateurStepperMotor"(reference=w444, "Position"=w443) -> (reference out=w442:refnum<k24>)  [unwired: 1 in, 1 out]
            n207 = property class="AmateurStepperMotor"(reference=w442) -> ("Position"=w441:dbl)  [unwired: 1 in, 2 out]
            n208 = local write "Position"(w441) -> ()
          }
        }
      }
      event "Стоп": Value Change {
        n209 = event-data() -> ()  [unwired: 1 in, 6 out]
        n210 = local read "Стоп"() -> (w445:bool)
      }
    }
  }
  n211 = while {
    shift-right: [w448] -> _
    shift-left: 0 -> [w449]
    tunnel: w39 -> [_]
    stop <- w452 stop-if-true
    # "Управление Ардуино тумблерами"
    n212 = local read "Стоп"() -> (w452:bool)
    n213 = Wait (ms)(milliseconds to wait=u32 10 ("millisecond timer value")) -> ()  [unwired: 1 out]
    n214 = Boolean Array To Number(Boolean array="Сегменты") -> (number=w447:u32)
    n215 = To Long Integer(number=w447) -> (32bit integer=w448:i32)
    n216 = Not Equal?(x=w448, y=w449) -> (x != y?=w450:bool)
    n217 = case shown="True" w450 {
      tunnel: w448 -> [_ w453]
      tunnel: w449 -> [_ w454]
      frame False {
      }
      frame True {
        n218 = stacked-sequence {
          seq-local: [w457 _ _] -> [_ w468 _]
          seq-local: [w455 _ _] -> [_ w463 _]
          seq-local: [_ w464 _] -> [_ _ w504]
          tunnel: w453 -> [w459 _ _]
          tunnel: w454 -> [w458 _ _]
          frame #0 {
            # "Детектирвоание позиции и\nнаправления изменения бита"
            n219 = Subtract(x=w459, y=w458) -> (x-y=w460:i32)
            n220 = To Double Precision Float(number=w460) -> (double precision float=w461:dbl)
            n221 = Greater Than 0?(x=w460) -> (x > 0?=w457:bool)
            "+/-" <- w457
            n222 = Absolute Value(x=w461) -> (abs(x)=w456:dbl)
            n223 = Logarithm Base 2(1:w456) -> (0:w455:dbl)
            "Разряд" <- w455
          }
          frame #1 {
            # "Указывает на последнюю нажатую кнопку"
            # "Выбор бита и направления\n его измнения"
            n224 = case shown="10" w463 {
              tunnel: ["D10" "D9" "D5" "D8" "D11" "D12" "A1" "D4" "A5" "A4" "A3" "A2" "A0" "D13" "D3" "All"] -> w466
              tunnel: ["a" "b" "c" "d" "e" "f" "g" "h" "j" "k" "L" "m" "n" "p" "dp" "All"] -> w462
              frame 0, Default {
                # "a = D10"
              }
              frame 1 {
                # "b = D9"
              }
              frame 2 {
                # "c = D5"
              }
              frame 3 {
                # "d = D8"
              }
              frame 4 {
                # "e = D11"
              }
              frame 5 {
                # "f = D12"
              }
              frame 6 {
                # "g = A1"
              }
              frame 7 {
                # "h = D4"
              }
              frame 8 {
                # "j = A5"
              }
              frame 9 {
                # "k = A4"
              }
              frame 10 {
                # "L = A3"
              }
              frame 11 {
                # "m = A2"
              }
              frame 12 {
                # "n = A0"
              }
              frame 13 {
                # "p = D13"
              }
              frame 14 {
                # "dp = D3"
              }
              frame 15 {
              }
            }
            "Сегмент" <- w462
            n225 = Select(t="off", s=w468, f="on") -> (s? t:f=w465:string)
            n226 = Concatenate Strings(w466, "_" ("string"), w465) -> (w464:string)
          }
          frame #2 {
            # "Передача команды в Ардуино"
            n227 = Equal?(x=w504, y="All_off") -> (x = y?=w507:bool)
            n228 = Equal?(x=w504, y="All_on") -> (x = y?=w505:bool)
            n229 = case shown="True" w507 {
              frame False {
              }
              frame True {
                n230 = local write "Сегменты"(bool[] [TRUE, TRUE, TRUE, TRUE, TRUE, TRUE, TRUE, TRUE, TRUE, TRUE, TRUE, TRUE, TRUE, TRUE, TRUE, TRUE] ("Сегменты")) -> ()
              }
            }
            n231 = case shown="True" w505 {
              frame False {
              }
              frame True {
                n232 = local write "Сегменты"(bool[] [FALSE, FALSE, FALSE, FALSE, FALSE, FALSE, FALSE, FALSE, FALSE, FALSE, FALSE, FALSE, FALSE, FALSE, FALSE, FALSE] ("Сегменты")) -> ()
              }
            }
            n233 = stacked-sequence {
              tunnel: w504 -> [w510 _ _]
              frame #0 {
                n234 = local write "Command"(w510) -> ()
              }
              frame #1 {
                n235 = local write "Записать"(TRUE ("Записать")) -> ()
                n236 = Wait (ms)(milliseconds to wait=u32 1000) -> ()  [unwired: 1 out]
              }
              frame #2 {
                n237 = local write "Записать"(FALSE ("Записать")) -> ()
                n238 = Wait (ms)(milliseconds to wait=u32 1000) -> ()  [unwired: 1 out]
              }
            }
          }
        }
      }
    }
  }
  n239 = call <instrlib>:"niDMM Close.vi"("error in (no error)"=w32, "instrument handle"=w33) -> ()  [unwired: 9 in, 1 out]
  n240 = while {
    tunnel: [w521] -> w34
    tunnel: w37 -> [w519]
    tunnel: w36 -> [w518]
    tunnel: [w515] -> w35
    stop <- w517 stop-if-true
    # "Настройка вольтметра NI PXI-4071"
    n241 = Wait (ms)(milliseconds to wait=u32 1) -> ()  [unwired: 1 out]
    n242 = flat-sequence {
      tunnel: [w528] -> w523
      tunnel: w519 -> [w526]
      tunnel: w518 -> [w530]
      tunnel: [w527] -> w522
      tunnel: w523 -> [w539]
      tunnel: w522 -> [w542]
      tunnel: [w538] -> w517
      tunnel: [w537] -> w515
      tunnel: [w536] -> w516
      frame #0 {
        w524 = T6 6.5 items=["3 1/2"=3.5, "4 1/2"=4.5, "5 1/2"=5.5, "6 1/2"=6.5, "7 1/2"=7.5] ("Resolution in Digits")
        n243 = Fract/Exp String To Number(string="NI DMM 1 Voltage Range 4") -> (number=w529:dbl)  [unwired: 3 in, 1 out]
        n244 = call-poly <instrlib>:"niDMM Config Measurement.vi"("Range"=w529, "Resolution in Digits"=w524, "error in (no error)"=w530, "Function"=niDMM_Function."DC Volts" ("Measurement Type"), "instrument handle"=w526) -> ("error out"=w527:errorcluster, "instrument handle out"=w528:refnum<k15>)  [unwired: 5 in]
      }
      frame #1 {
        n245 = call <instrlib>:"niDMM Read.vi"("error in (no error)"=w542, "instrument handle"=w539) -> ("error out"=w536:errorcluster, "Measurement"=w534:dbl, "instrument handle out"=w537:refnum<k15>)  [unwired: 7 in]
        "Voltage, V" <- w534
        n246 = Fract/Exp String To Number(string="NI DMM 1 units 4") -> (number=w540:dbl)  [unwired: 3 in, 1 out]
        n247 = Multiply(x=w540, y=w534) -> (x*y=w532:dbl)
        n248 = Absolute Value(x=w532) -> (abs(x)=→"Voltage Char":dbl)
        n249 = Absolute Value(x=w532) -> (abs(x)=→"Voltage":dbl)
        n250 = local read "Стоп"() -> (w538:bool)
      }
    }
    n251 = call <vilib>:"Simple Error Handler.vi"("error in (no error)"=w516) -> ("error out"=w521:errorcluster)  [unwired: 1 in, 7 out]
  }
  n252 = invoke class="AmateurStepperMotor" method="Stop"(reference=w7) -> (reference out=w14:refnum<k24>, "Stop"=w15:refnum<k24>)  [unwired: 2 in, 1 out]
  n253 = property class="AmateurStepperMotor"(reference=w14, "HoldOn"=FALSE) -> (reference out=w13:refnum<k24>)  [unwired: 1 in, 1 out]
  n254 = invoke class="AmateurStepperMotor" method="Dispose"(reference=w13) -> (error out=w10:errorcluster)  [unwired: 2 in, 2 out]
  n255 = invoke class="SerialPort" method="Close"(reference=w25, error in=w10) -> (reference out=w9:refnum<k24>, error out=w11:errorcluster)  [unwired: 1 in, 1 out]
  n256 = invoke class="Task" method="Wait"(reference=w15) -> ()  [unwired: 2 in, 3 out]
  n257 = Close Reference(reference=w9, error in (no error)=w11) -> (error out=w12:errorcluster)
  n258 = call <vilib>:"Simple Error Handler.vi"("error in (no error)"=w12) -> ()  [unwired: 1 in, 8 out]
  n259 = VISA Close(VISA resource name=w18, error in (no error)=w17) -> (error out=w27:errorcluster)
  n260 = call <instrlib>:"niDMM Close.vi"("error in (no error)"=w34, "instrument handle"=w35) -> ()  [unwired: 9 in, 1 out]
  n261 = call <instrlib>:"niDCPower Close.vi"("instrument handle"=w40) -> ()  [unwired: 10 in, 1 out]
  n262 = call "Ophir Error Message.vi"("error in (no error)"=w27) -> ()  [unwired: 3 in, 4 out]
